vi "ConvertArrayToMessages.vi"(8 "error in (no error)":errorcluster, 11 "Array":bool[][](array[boolean])=array64x128[8192 elements]) -> (0 "error out":errorcluster, 3 "Messages":string[](array[string]))   [LabVIEW 2024, in "OLEDI2CMessageGenerator.lvlib"]
uses:
  OLEDI2CMessageGenerator.lvlib
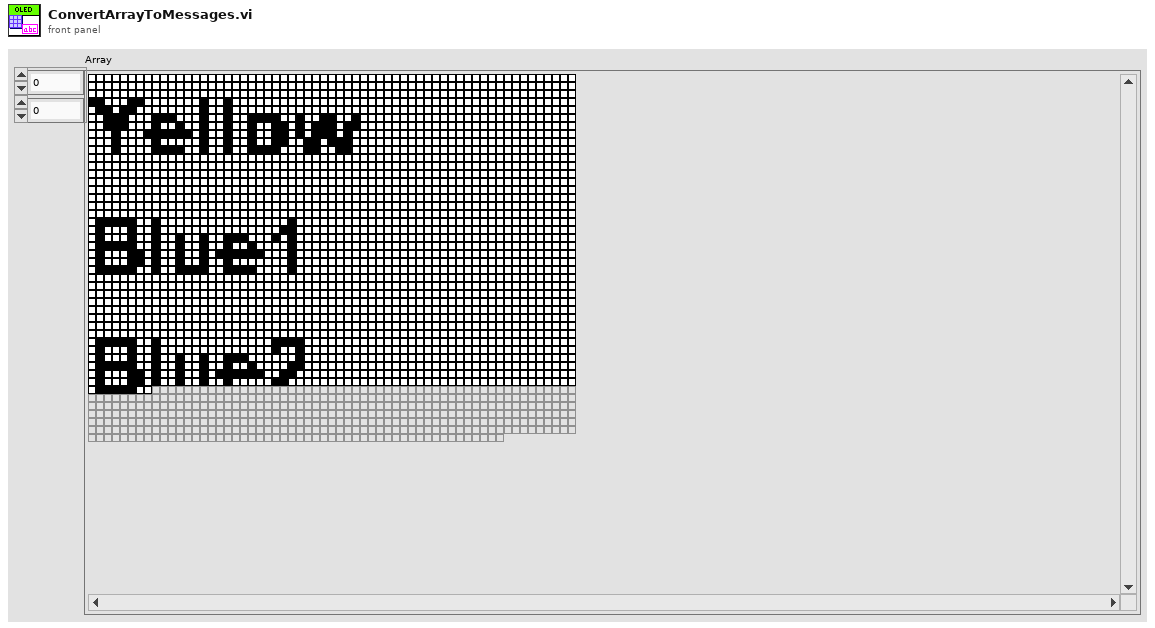
[diagram p1: front panel]
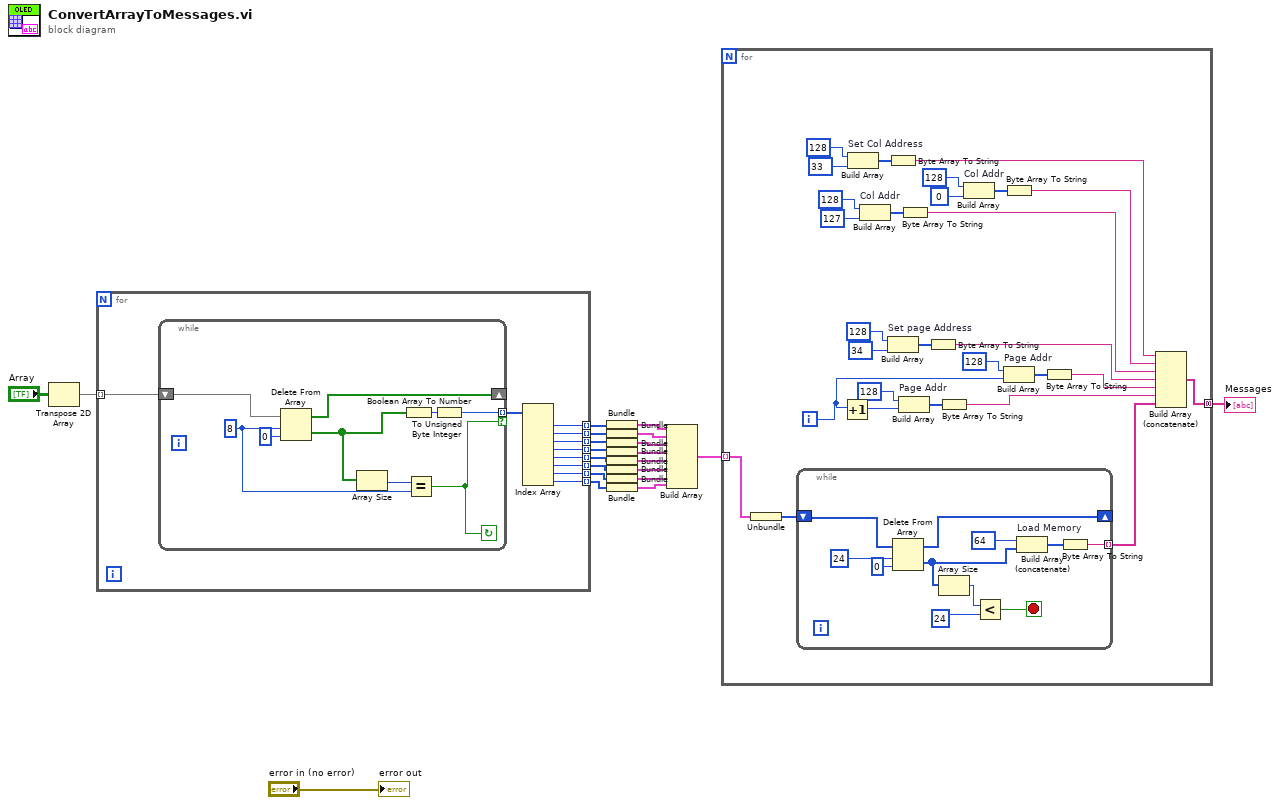
[diagram p0: block diagram]
diagram:
  n1 = Transpose 2D Array(2D array="Array") -> (transposed array=w20:bool[][])
  n2 = for {
    tunnel: w20 -> [w22] mode=indexing
    tunnel: [w30] -> w19 mode=indexing
    tunnel: [w29] -> w18 mode=indexing
    tunnel: [w28] -> w17 mode=indexing
    tunnel: [w27] -> w16 mode=indexing
    tunnel: [w26] -> w15 mode=indexing
    tunnel: [w25] -> w14 mode=indexing
    tunnel: [w24] -> w13 mode=indexing
    tunnel: [w23] -> w12 mode=indexing
    n3 = while {
      shift-right: [w36] -> _
      shift-left: w22 -> [w37]
      tunnel: [w40] -> w31 mode=indexing if=w32
      stop <- w32 continue-if-true
      w33 = 8 ("y")
      n4 = Delete From Array(array=w37, length=w33, index=0) -> (deleted portion=w35:bool[], array with subset deleted=w36:bool[])
      n5 = Array Size(array=w35) -> (size(s)=w34:i32)
      n6 = Boolean Array To Number(Boolean array=w35) -> (number=w39:u32)
      n7 = Equal?(x=w34, y=w33) -> (x = y?=w32:bool)
      n8 = To Unsigned Byte Integer(number=w39) -> (unsigned 8bit integer=w40:u8)
    }
    n9 = Index Array(array=w31) -> (element #1=w30:u8, element #2=w29:u8, element #3=w28:u8, element #4=w27:u8, element #5=w26:u8, element #6=w25:u8, element #7=w24:u8, element #8=w23:u8)  [unwired: 8 in]
  }
  n10 = Bundle(w19) -> (w11:cluster{u8[]})  [unwired: 1 in]
  n11 = Bundle(w18) -> (w10:cluster{u8[]})  [unwired: 1 in]
  n12 = Bundle(w17) -> (w9:cluster{u8[]})  [unwired: 1 in]
  n13 = Bundle(w16) -> (w8:cluster{u8[]})  [unwired: 1 in]
  n14 = Bundle(w15) -> (w7:cluster{u8[]})  [unwired: 1 in]
  n15 = Bundle(w14) -> (w6:cluster{u8[]})  [unwired: 1 in]
  n16 = Bundle(w13) -> (w5:cluster{u8[]})  [unwired: 1 in]
  n17 = Bundle(w12) -> (w4:cluster{u8[]})  [unwired: 1 in]
  n18 = Build Array(w11, w10, w9, w8, w7, w6, w5, w4) -> (w2:cluster{u8[]}[])
  n19 = for {
    tunnel: [w68] -> w3 mode=concatenating
    tunnel: w2 -> [w67] mode=indexing
    i -> [w56]
    n20 = Unbundle(w67) -> (w66:u8[])
    n21 = while {
      shift-right: [w76] -> _
      shift-left: w66 -> [w78]
      tunnel: [w70] -> w65 mode=indexing
      stop <- w72 stop-if-true
      n22 = Delete From Array(array=w78, length=24 ("y"), index=0) -> (deleted portion=w74:u8[], array with subset deleted=w76:u8[])
      n23 = Array Size(array=w74) -> (size(s)=w73:i32)
      n24 = Less?(x=w73, y=24) -> (x < y?=w72:bool)
      n25 = Build Array (concatenate) "Load Memory"(u8 64 ("element"), w74) -> (w71:u8[])
      n26 = Byte Array To String(unsigned byte array=w71) -> (string=w70:string)
    }
    n27 = Increment(x=w56) -> (x+1=w57:i32)
    n28 = Build Array "Set Col Address"(u8 128 ("element"), u8 33 ("element")) -> (w50:u8[])
    n29 = Build Array "Col Addr"(u8 128 ("element"), u8 127 ("element")) -> (w44:u8[])
    n30 = Byte Array To String(unsigned byte array=w50) -> (string=w41:string)
    n31 = Build Array "Set page Address"(u8 128 ("element"), u8 34 ("element")) -> (w62:u8[])
    n32 = Build Array "Page Addr"(u8 128 ("element"), w57) -> (w58:i32[])
    n33 = Byte Array To String(unsigned byte array=w44) -> (string=w43:string)
    n34 = Byte Array To String(unsigned byte array=w62) -> (string=w55:string)
    n35 = Byte Array To String(unsigned byte array=w58) -> (string=w53:string)
    n36 = Build Array "Col Addr"(u8 128 ("element"), u8 0 ("element")) -> (w49:u8[])
    n37 = Byte Array To String(unsigned byte array=w49) -> (string=w42:string)
    n38 = Build Array "Page Addr"(u8 128 ("element"), w56) -> (w61:i32[])
    n39 = Byte Array To String(unsigned byte array=w61) -> (string=w54:string)
    n40 = Build Array (concatenate)(w41, w42, w43, w55, w54, w53, w65) -> (w68:string[])
  }
  "Messages" <- w3
  "error out" <- "error in (no error)"
